vi "write_data_to_temp_file.vi"(2 "error in (no error)":errorcluster, 3 "Data Array":T1(array[cluster])) -> (0 "error out":errorcluster)   [LabVIEW 2010]
uses:
  <vilib>/Utility/xml.llb/Write to XML File(string).vi
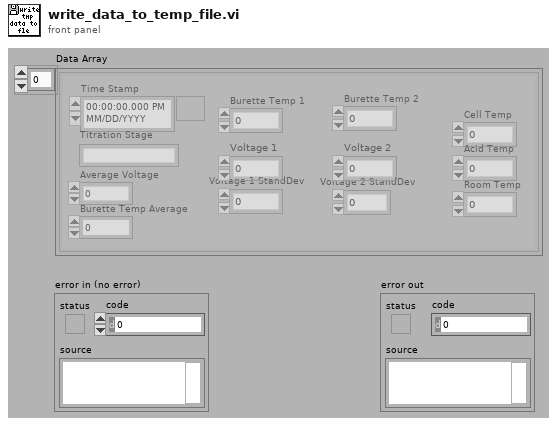
[diagram p1: front panel]
types:
  T1 = cluster{"Time Stamp":timestamp, "Titration Stage":string, "Average Voltage":dbl, "Burette Temp Average":dbl, "Voltage 1":dbl, "Voltage 2":dbl, "Voltage 1 StandDev":dbl, "Voltage 2 StandDev":dbl, "Burette Temp 1":dbl, "Burette Temp 2":dbl, "Cell Temp":dbl, "Acid Temp":dbl, "Room Temp":dbl}[]
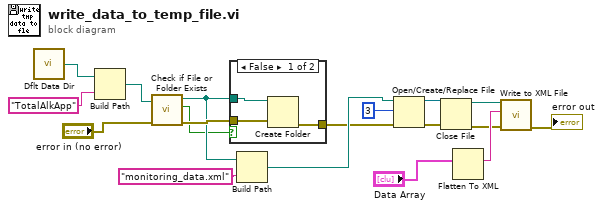
[diagram p0: block diagram]
diagram:
  n1 = call <vilib>:"Dflt Data Dir.vi"() -> ("App:Default Data Directory"=w6:path)
  n2 = Build Path(base path=w6, name or relative path="TotalAlkApp") -> (appended path=w9:path)
  n3 = call <vilib>:"Check if File or Folder Exists.vi"("error in (no error)"="error in (no error)", "path"=w9) -> ("error out"=w10:errorcluster, "file or folder exists?"=w1:bool, "dup path"=w2:path)  [unwired: 7 in]
  n4 = case shown="False" w1 {
    tunnel: w2 -> [w21 _]
    tunnel: w10 -> [w20 w22]
    tunnel: [w19 w22] -> w14
    frame False {
      n5 = Create Folder(path (use dialog)=w21, error in=w20) -> (error out=w19:errorcluster)  [unwired: 1 in, 2 out]
    }
    frame True {
    }
  }
  n6 = Build Path(base path=w2, name or relative path="monitoring_data.xml") -> (appended path=w15:path)
  n7 = Open/Create/Replace File(file path (use dialog)=w15, error in=w14, operation (0:open)=3) -> (refnum out=w12:refnum<file>, error out=w11:errorcluster)  [unwired: 3 in, 1 out]
  n8 = Close File(refnum=w12, error in=w11) -> (path=w4:path, error out=w5:errorcluster)
  n9 = Flatten To XML(anything="Data Array") -> (xml string=w18:string)
  n10 = call-poly <vilib>:"Write to XML File.vi"("error in (no error)"=w5, "XML Input"=w18, "XML File Path"=w4) -> ("error out"=→"error out":errorcluster)  [unwired: 6 in, 2 out]
